vi "Post-Build Action ErrorFiles.vi"(5 "Files Generated by Build":path[](array[path]), 6 "Top Level/Always Included VIs":path[](array[path]), 7 "Destination Path":path, 8 "error in (no error)":errorcluster, 9 "Target Name":string, 10 "Build Specification Name":string, 11 "Project Path":path) -> (0 "error out":errorcluster)   [LabVIEW 2020]
uses:
  <vilib>/Utility/sysdir.llb/System Directory Type.ctl
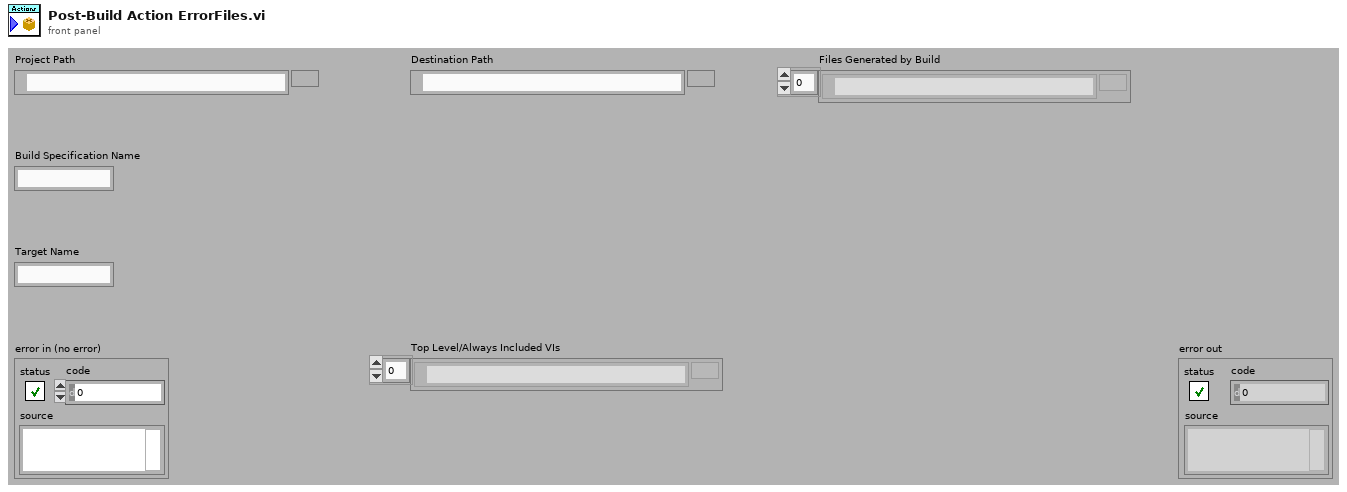
[diagram p1: front panel]
types:
  T1 = typedef "System Directory Type.ctl" = i32
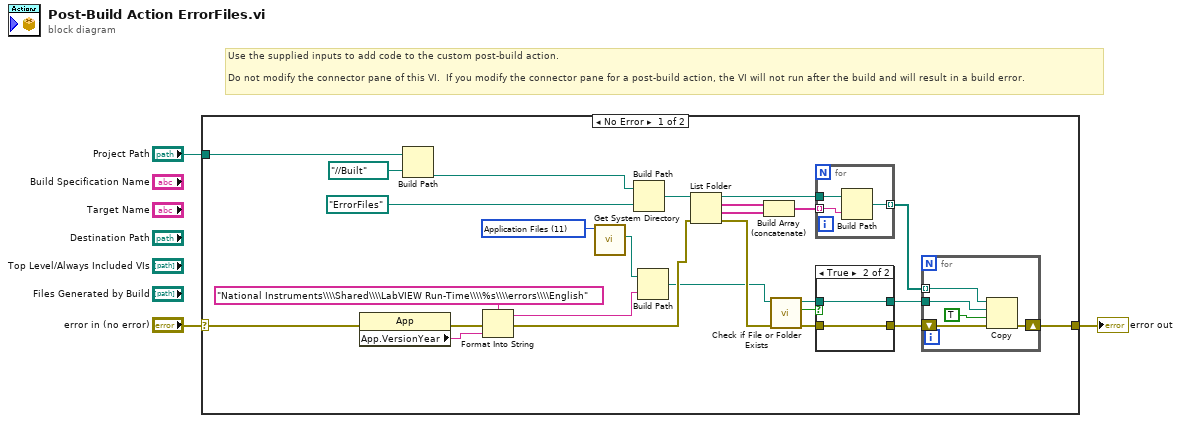
[diagram p0: block diagram]
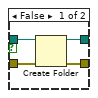
[diagram p2: hidden frame]
diagram:
  # "Use the supplied inputs to add code to the custom post-build action.\n\nDo not modify the connector pane of this VI.  If you modify the connector pane for a post-build action, the VI will not run after the build and will result in a build error."
  n1 = case shown="No Error" "error in (no error)" {
    selector: "error in (no error)" -> [w6 w44]
    tunnel: [w17 w44] -> w3
    tunnel: "Project Path" -> [w21 _]
    frame No Error {
      w8 = T1 11 items=["User Home"=0, "User Desktop"=1, "User Documents"=2, "User Application Data"=3, "User Preferences"=4, "User Temporary"=5, "Public Documents"=6, "Public Application Data"=7, "Public Preferences"=8, "Public Cache"=13, "System Core Libraries"=9, "System Installed Libraries"=10, "Application Files"=11, "Boot Volume Root"=12] ("system directory type")
      n2 = property class="App"(error in=w6) -> (error out=w11:errorcluster, "App.VersionYear"=w12:string)  [unwired: 1 in, 1 out]
      n3 = Build Path(base path=w21, name or relative path=path "../../Built") -> (appended path=w23:path)
      n4 = Format Into String(format string="National Instruments\\\\Shared\\\\LabVIEW Run-Time\\\\%s\\\\errors\\\\English" ("name or relative path"), error in=w11, w12) -> (resulting string=w9:string, error out=w5:errorcluster)  [unwired: 1 in]
      n5 = call <vilib>:"Get System Directory.vi"("system directory type"=w8) -> ("system directory"=w10:path)  [unwired: 10 in]
      n6 = Build Path(base path=w23, name or relative path=path "ErrorFiles") -> (appended path=w25:path)
      n7 = Build Path(base path=w10, name or relative path=w9) -> (appended path=w4:path)
      n8 = List Folder(path=w25, error in=w5) -> (path out=w26:path, filenames=w15:string[], folder names=w16:string[], error out=w24:errorcluster)  [unwired: 2 in]
      n9 = Build Array (concatenate)(w15, w16) -> (w14:string[])
      n10 = call <vilib>:"Check if File or Folder Exists.vi"("error in (no error)"=w24, "path"=w4) -> ("error out"=w27:errorcluster, "file or folder exists?"=w29:bool, "dup path"=w28:path)  [unwired: 7 in]
      n11 = for {
        tunnel: w14 -> [w42] mode=indexing
        tunnel: w26 -> [w43]
        tunnel: [w41] -> w13 mode=indexing
        n12 = Build Path(base path=w43, name or relative path=w42) -> (appended path=w41:path)
      }
      n13 = case shown="True" w29 {
        tunnel: w28 -> [w33 w35]
        tunnel: w27 -> [w32 w34]
        tunnel: [w31 w35] -> w19
        tunnel: [w30 w34] -> w20
        frame False {
          n14 = Create Folder(path (use dialog)=w33, error in=w32) -> (created path=w31:path, error out=w30:errorcluster)  [unwired: 1 in, 1 out]
        }
        frame True {
        }
      }
      n15 = for {
        tunnel: w13 -> [w37] mode=indexing
        shift-right: [w38] -> w17
        shift-left: w20 -> [w39]
        tunnel: w19 -> [w36]
        n16 = Copy(8:w39, 9:TRUE ("overwrite (F)"), 10:w36, 11:w37) -> (0:w38:errorcluster)  [unwired: 1 in, 2 out]
      }
    }
    frame Error {
    }
  }
  "error out" <- w3
